vi "CtrlTreePathsOfVI.vi"(10 "Selection":string[](array[string]), 11 "TreeControl in":refnum<vi>) -> (2 "VI List":string[](array[string]), 3 "App List":string[](array[string]))   [LabVIEW 2021]
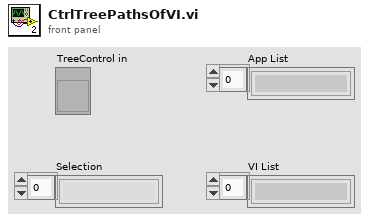
[diagram p1: front panel]
types:
  T1 = map{string, cluster{"Path":string, "application reference":refnum<vi>}}
  T2 = cluster{"Path":string, "application reference":refnum<vi>}
  T3 = cluster{"string array[0]":string, "string array[1]":string, "string array[2]":string, "string array[3]":string}
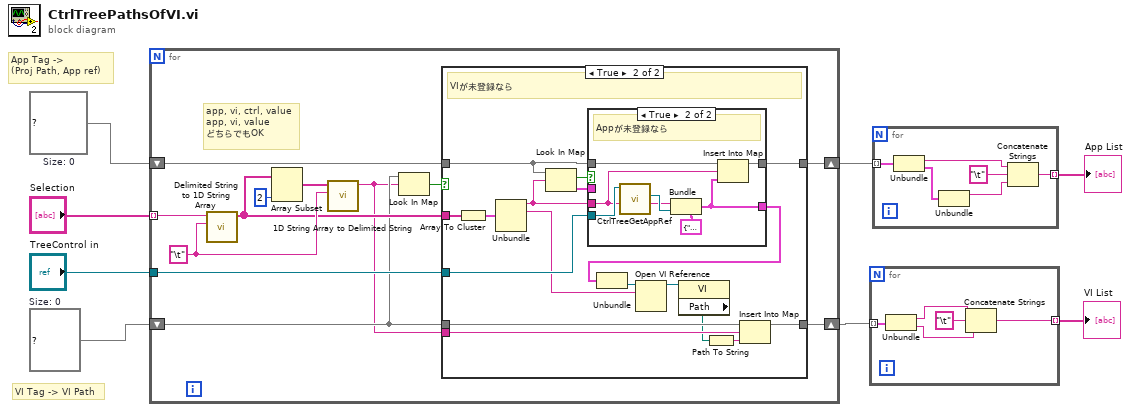
[diagram p0: block diagram]
diagram:
  w5 = map{string, string} {}  # Size: 0
  w7 = T1 {}  # Size: 0
  # "App Tag -> \n(Proj Path, App ref)"
  # "VI Tag -> VI Path"
  n1 = for {
    tunnel: "Selection" -> [w20] mode=indexing
    shift-right: [w17] -> w3
    shift-left: w7 -> [w18]
    tunnel: "TreeControl in" -> [w19]
    shift-right: [w9] -> w4
    shift-left: w5 -> [w11]
    w16 = "\t" ("delimiter")
    # "app, vi, ctrl, value\napp, vi, value\nどちらでもOK"
    n2 = call <vilib>:"Delimited String to 1D String Array.vi"("delimiter"=w16, "delimited string"=w20) -> ("string array"=w14:string[])  [unwired: 9 in]
    n3 = Array Subset(array=w14, length=2) -> (w13:string[])  [unwired: 1 in]
    n4 = call <vilib>:"1D String Array to Delimited String.vi"("delimiter"=w16, "string array"=w13) -> ("delimited string"=w10:string)  [unwired: 9 in]
    n5 = Look In Map(map=w11, key=w10) -> (key not found?=w12:bool)  [unwired: 1 in, 1 out]
    n6 = case shown="True" w12 {
      tunnel: w19 -> [_ w37]
      tunnel: w18 -> [w22 w35]
      tunnel: [w22 w34] -> w17
      tunnel: w14 -> [_ w33]
      tunnel: w11 -> [w21 w29]
      tunnel: w10 -> [_ w28]
      tunnel: [w21 w25] -> w9
      frame False {
      }
      frame True {
        # "VIが未登録なら"
        n7 = Array To Cluster(array=w33) -> (cluster=w39:T3)
        n8 = Unbundle(w39) -> ("string array[0]"=w36:string, "string array[1]"=w31:string)  [unwired: 2 out]
        n9 = Look In Map(map=w35, key=w36) -> (key not found?=w38:bool, value=w32:T2)  [unwired: 1 in]
        n10 = case shown="True" w38 {
          tunnel: w37 -> [_ w49]
          tunnel: w36 -> [_ w47]
          tunnel: w35 -> [w41 w48]
          tunnel: [w41 w46] -> w34
          tunnel: w32 -> [w40 _]
          tunnel: [w40 w42] -> w24
          frame False {
          }
          frame True {
            # "Appが未登録なら"
            n11 = call "CtrlTreeGetAppRef.vi"("App Tag"=w47, "ControlTree in"=w49) -> ("Path"=w43:string, "Application out"=w44:refnum<vi>)  [unwired: 6 in, 2 out]
            n12 = Bundle(cluster=T2 {"Path"="", "application reference"=refnum}, "Path"=w43, "application reference"=w44) -> (w42:T2)
            n13 = Insert Into Map(map in=w48, key=w47, value=w42) -> (map out=w46:T1)  [unwired: 2 out]
          }
        }
        n14 = Unbundle(w24) -> ("application reference"=w23:refnum<vi>)  [unwired: 1 out]
        n15 = Open VI Reference(application reference (local)=w23, vi path=w31) -> (vi reference=w30:refnum<vi>)  [unwired: 4 in, 1 out]
        n16 = property class="VI"(reference=w30) -> ("Path"=w26:path)  [unwired: 1 in, 2 out]
        n17 = Path To String(path=w26) -> (string=w27:string)
        n18 = Insert Into Map(map in=w29, key=w28, value=w27) -> (map out=w25:map{string, string})  [unwired: 2 out]
      }
    }
  }
  n19 = for {
    tunnel: w4 -> [w54] mode=indexing
    tunnel: [w50] -> w2 mode=indexing
    n20 = Unbundle(w54) -> (w52:string, w51:string)
    n21 = Concatenate Strings(w52, "\t" ("string"), w51) -> (w50:string)
  }
  "VI List" <- w2
  n22 = for {
    tunnel: w3 -> [w60] mode=indexing
    tunnel: [w55] -> w1 mode=indexing
    n23 = Unbundle(w60) -> (w56:string, w59:T2)
    n24 = Unbundle(w59) -> ("Path"=w57:string)  [unwired: 1 out]
    n25 = Concatenate Strings(w56, "\t" ("string"), w57) -> (w55:string)
  }
  "App List" <- w1
